vi "LDT Telescope Obs Status FG.vi"(10 "Write?":bool, 11 "String":string) -> (2 "Timestamp":timestamp, 3 "status string out":string)   [LabVIEW 2022 SP3, in "LDT Telescope.lvclass"]
uses:
  LDT Telescope.lvclass
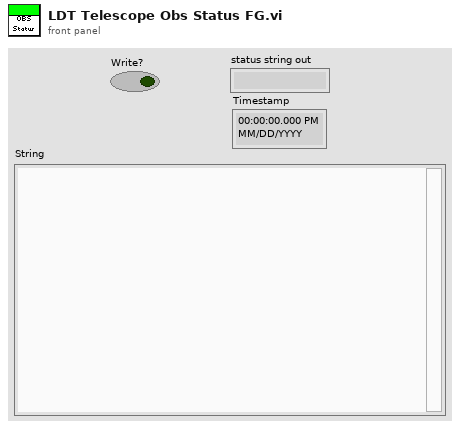
[diagram p1: front panel]
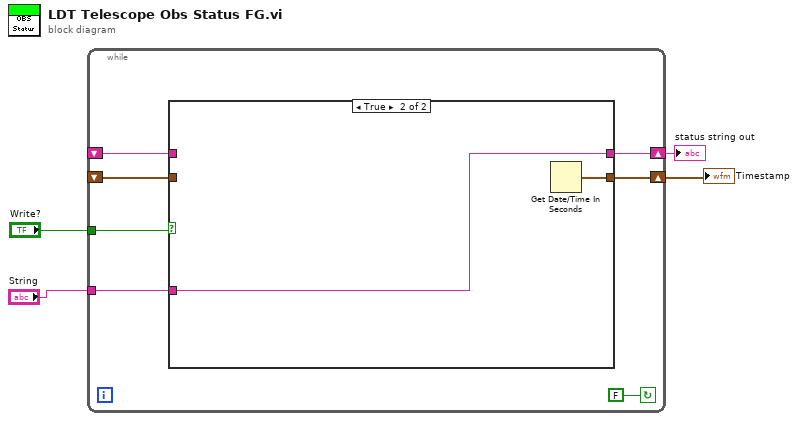
[diagram p0: block diagram]
diagram:
  n1 = while {
    shift-right: [w10] -> w2
    shift-left: _ -> [w6]
    tunnel: "Write?" -> [w11]
    shift-right: [w8] -> w1
    shift-left: _ -> [w5]
    tunnel: "String" -> [w9]
    stop <- FALSE continue-if-true
    n2 = case shown="True" w11 {
      tunnel: [w13 w15] -> w10
      tunnel: w9 -> [_ w15]
      tunnel: [w12 w14] -> w8
      tunnel: w6 -> [w13 _]
      tunnel: w5 -> [w12 _]
      frame False {
      }
      frame True {
        n3 = Get Date/Time In Seconds() -> (seconds since 1Jan1904=w14:timestamp)
      }
    }
  }
  "status string out" <- w2
  "Timestamp" <- w1
